vi "Initialize-object.vi"(8 "error in":errorcluster, 10 "Main VI ref":refnum<vi>) -> (0 "error IO":errorcluster, 3 "UI ref.":refnum<data-value>)   [LabVIEW 2013, in "CameraVision.lvlib" / "CV-UI.lvclass"]
doc: "This function deletes the data from the various GUI graphs and displays. This avoids interference with data from a previous acquisition."
uses:
  CV-UI.lvclass
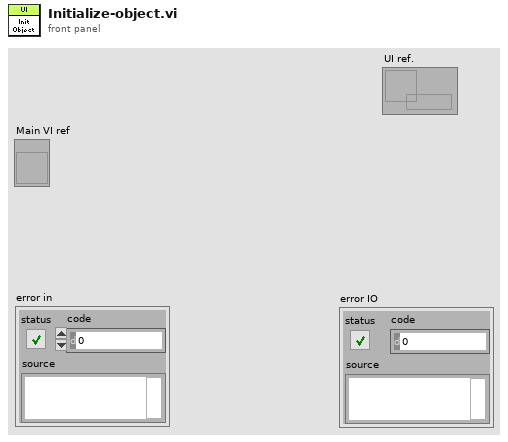
[diagram p1: front panel]
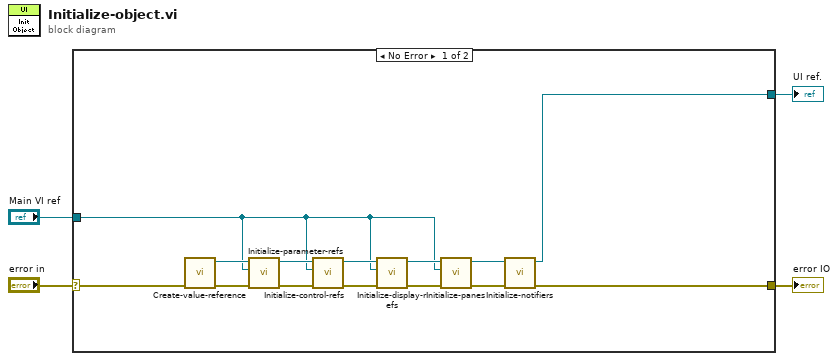
[diagram p0: block diagram]
diagram:
  n1 = case shown="No Error" "error in" {
    selector: "error in" -> [w18 w19]
    tunnel: [w17 w19] -> w4
    tunnel: [w10 _] -> w2
    tunnel: "Main VI ref" -> [w7 _]
    frame No Error {
      n2 = call "Create-value-reference.vi"("error in (no error)"=w18) -> ("error out"=w16:errorcluster, "UI ref."=w11:refnum<data-value>)  [unwired: 9 in]
      n3 = call "Initialize-parameter-refs.vi"("error in (no error)"=w16, "VI ref"=w7, "UI ref. in"=w11) -> ("error out"=w14:errorcluster, "UI ref."=w15:refnum<data-value>)  [unwired: 7 in]
      n4 = call "Initialize-control-refs.vi"("error in (no error)"=w14, "VI ref"=w7, "UI ref. in"=w15) -> ("error out"=w12:errorcluster, "UI ref."=w13:refnum<data-value>)  [unwired: 7 in]
      n5 = call "Initialize-display-refs.vi"("error in (no error)"=w12, "VI ref"=w7, "UI ref. in"=w13) -> ("error out"=w8:errorcluster, "UI ref."=w9:refnum<data-value>)  [unwired: 7 in]
      n6 = call "Initialize-panes.vi"("error in (no error)"=w8, "VI ref"=w7, "UI ref. in"=w9) -> ("error out"=w5:errorcluster, "UI ref."=w6:refnum<data-value>)  [unwired: 7 in]
      n7 = call "Initialize-notifiers.vi"("error in (no error)"=w5, "UI ref. in"=w6) -> ("error out"=w17:errorcluster, "UI ref."=w10:refnum<data-value>)  [unwired: 8 in]
    }
    frame Error {
    }
  }
  "error IO" <- w4
  "UI ref." <- w2
